vi "initialize.vi"(8 "error in (no error)":errorcluster, 11 "Agilent 34980A in":refnum<class "Agilent 34980A.lvclass">) -> (0 "error out":errorcluster, 1 "String Output":string, 2 "initialized?":bool, 3 "Agilent 34980A out":refnum<class "Agilent 34980A.lvclass">)   [LabVIEW 2017, in "Agilent 34980A.lvclass"]
doc: "Agilent:\ninitializes the Agilent unit"
uses:
  Agilent 34980A.lvclass
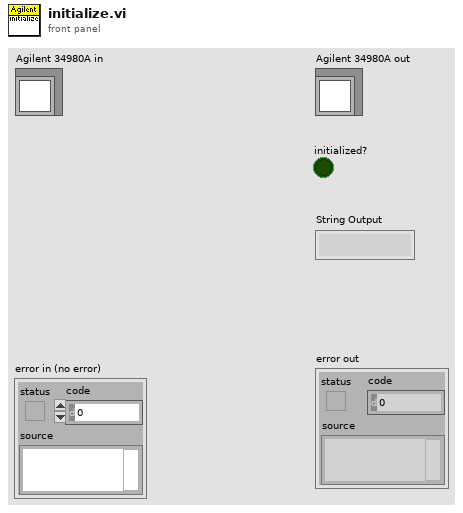
[diagram p1: front panel]
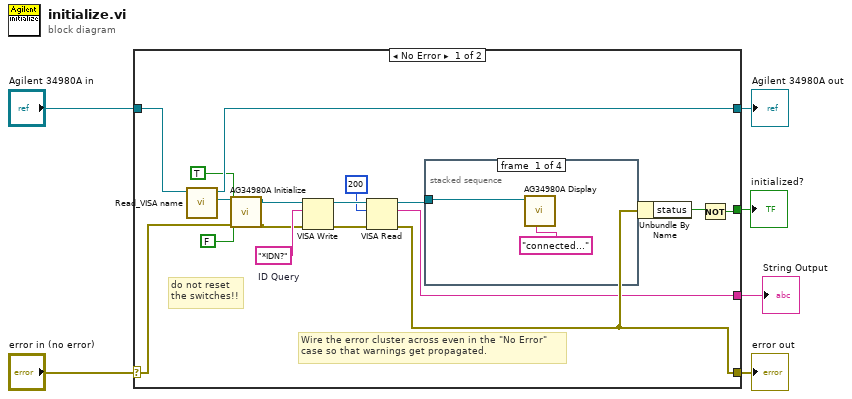
[diagram p0: block diagram]
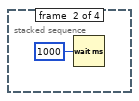
[diagram p2: hidden frame]
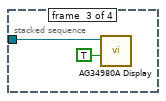
[diagram p3: hidden frame]
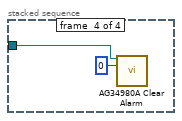
[diagram p4: hidden frame]
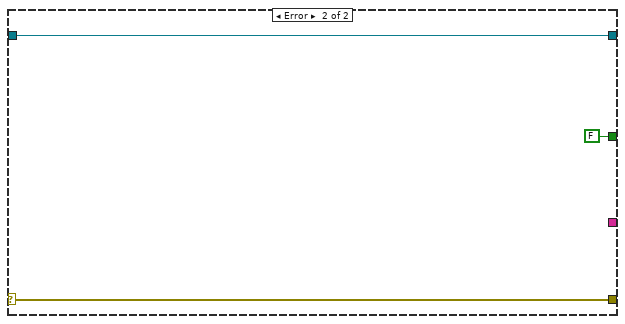
[diagram p5: hidden frame]
diagram:
  n1 = case shown="No Error" "error in (no error)" {
    selector: "error in (no error)" -> [w18 w33]
    tunnel: [w8 w33] -> w5
    tunnel: [w19 w32] -> w3
    tunnel: "Agilent 34980A in" -> [w20 w32]
    tunnel: [w22 FALSE ("status")] -> w2
    tunnel: [w7 _] -> w1
    frame No Error {
      w13 = "*IDN?"  # ID Query
      # "do not reset\nthe switches!!"
      # "Wire the error cluster across even in the \"No Error\"\ncase so that warnings get propagated."
      n2 = call-dynamic "Read_VISA name.vi"("instrument in"=w20) -> ("VISA resource name"=w21:refnum<visa-resource-name>, "instrument out"=w19:refnum<class "Agilent 34980A.lvclass">)  [unwired: 8 in, 1 out]
      n3 = call "AG34980A Initialize.vi"("VISA resource name"=w21, "ID Query (True)"=TRUE, "Reset (True)"=FALSE, "error in (no error)"=w18) -> ("VISA session"=w11:refnum<visa-resource-name>, "error out"=w10:errorcluster)  [unwired: 10 in]
      n4 = VISA Write(VISA resource name=w11, write buffer=w13, error in (no error)=w10) -> (VISA resource name out=w14:refnum<visa-resource-name>, error out=w15:errorcluster)  [unwired: 1 out]
      n5 = VISA Read(VISA resource name=w14, byte count=u32 200, error in (no error)=w15) -> (VISA resource name out=w9:refnum<visa-resource-name>, read buffer=w7:string, error out=w8:errorcluster)  [unwired: 1 out]
      n6 = stacked-sequence {
        tunnel: w9 -> [w24 _ w28 w30]
        frame #0 {
          n7 = call "AG34980A Display.vi"("Text to Display(empty)"="connected...", "VISA resource name"=w24) -> ()  [unwired: 6 in, 4 out]
        }
        frame #1 {
          n8 = Wait (ms)(milliseconds to wait=u32 1000) -> ()  [unwired: 1 out]
        }
        frame #2 {
          n9 = call "AG34980A Display.vi"("Clear Display (F:No)"=TRUE, "VISA resource name"=w28) -> ()  [unwired: 6 in, 4 out]
        }
        frame #3 {
          n10 = call "AG34980A Clear Alarm.vi"("VISA resource name"=w30, "Alarm Index (0: Clear All)"=0) -> ()  [unwired: 12 in, 2 out]
        }
      }
      n11 = Unbundle By Name(w8) -> ("status"=w23:bool)
      n12 = Not(x=w23) -> (.not. x?=w22:bool)
    }
    frame Error {
    }
  }
  "error out" <- w5
  "Agilent 34980A out" <- w3
  "initialized?" <- w2
  "String Output" <- w1
